vi "AIM_DataCollectAsCSV.vi"(5 "Data Reset?":bool, 7 "WRITE":bool, 10 "in X, Y Data":dbl[][](array[numeric]), 11 "Data File Name":string="Sample-Robot-2-Trajectory-TrajLibrary.csv") -> (0 "Y, X Pairs":T1[](array[typedef]) {"Y" format="%_7f"; "X" format="%_7f"}, 1 "X, Y Pairs":T1[](array[typedef]) {"Y" format="%_7f"; "X" format="%_7f"}, 2 "all Data":dbl[][](array[numeric]), 3 "Data File Name":string="Sample-Robot-2-Trajectory-TrajLibrary.csv")   [LabVIEW 2023]
uses:
  <vilib>/Rock Robotics/WPI/ThirdParty/JAS_Junk/TrajLib/TypeDef/X_Y_PAIR.ctl
  <vilib>/Utility/file.llb/Read Delimited Spreadsheet (DBL).vi
  <vilib>/Utility/file.llb/Write Delimited Spreadsheet (DBL).vi
  <vilib>/Rock Robotics/WPI/ThirdParty/JAS_Junk/TrajLib/Trajectory_Library.lvlib
panel:
  out "error out":errorcluster
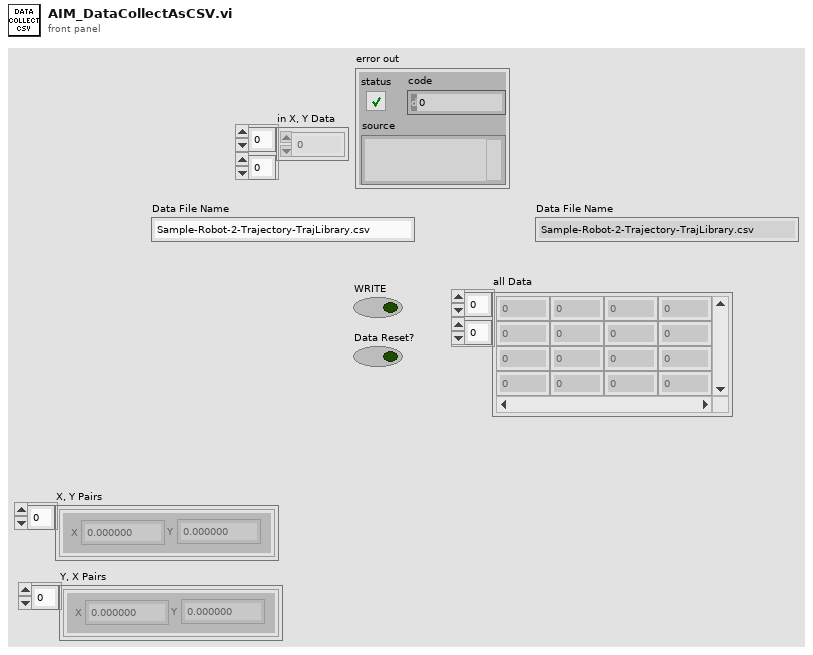
[diagram p1: front panel]
types:
  T1 = typedef "Trajectory_Library.lvlib/X_Y_PAIR.ctl" = cluster{"X":dbl, "Y":dbl}
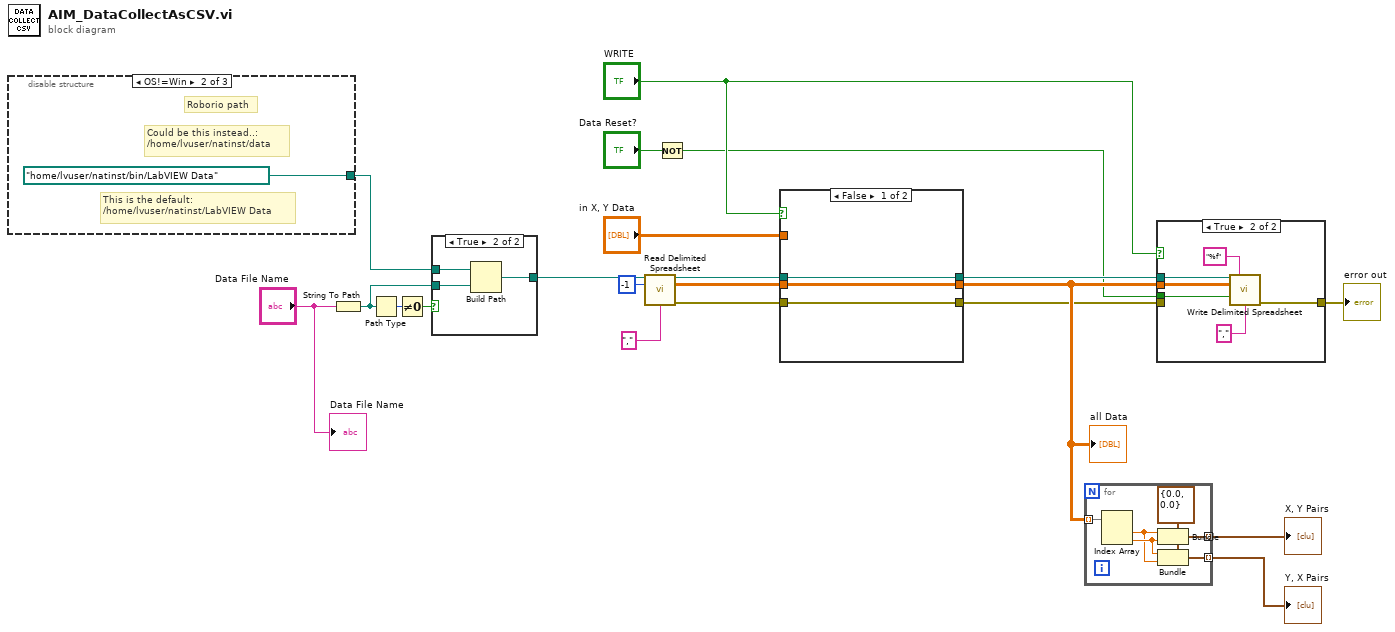
[diagram p0: block diagram]
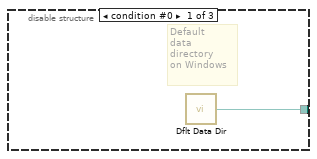
[diagram p4: hidden frame]
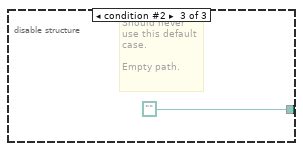
[diagram p5: hidden frame]
diagram:
  n1 = disable-structure shown="OS!=Win" {
    disable-tunnel: [w22 path "/home/lvuser/natinst/bin/LabVIEW Data" path ""] -> w19
    frame condition #0 {
      # "Default\ndata\ndirectory\non Windows"
      n2 = call <vilib>:"Dflt Data Dir.vi"() -> ("App:Default Data Directory"=w22:path)
    }
    frame condition #1 (active) {
      # "This is the default:\n/home/lvuser/natinst/LabVIEW Data"
      # "Could be this instead..:\n/home/lvuser/natinst/data"
      # "Roborio path"
    }
    frame condition #2 {
      # "Should never\nuse this default\ncase.\n\nEmpty path."
    }
  }
  n3 = String To Path(string="Data File Name") -> (path=w17:path)
  n4 = Path Type(1:w17) -> (0:w20:i16)
  n5 = Not Equal To 0?(x=w20) -> (x != 0?=w21:bool)
  n6 = case shown="True" w21 {
    tunnel: [w25 w28] -> w2
    tunnel: w19 -> [_ w27]
    tunnel: w17 -> [w25 w26]
    frame False {
    }
    frame True {
      n7 = Build Path(base path=w27, name or relative path=w26) -> (appended path=w28:path)
    }
  }
  n8 = call-poly <vilib>:"Read Delimited Spreadsheet.vi"("file path (dialog if empty)"=w2, "number of rows (all:-1)"=-1, "delimiter (\\t)"="," ("delimiter (\\t)")) -> ("new file path (Not A Path if cancelled)"=w1:path, "all rows"=w10:dbl[][], "error out"=w5:errorcluster)  [unwired: 7 in, 3 out]
  n9 = Not(x="Data Reset?") -> (.not. x?=w6:bool)
  n10 = case shown="False" "WRITE" {
    tunnel: w1 -> [w31 w34]
    tunnel: [w31 w34] -> w11
    tunnel: w10 -> [w30 _]
    tunnel: [w30 w33] -> w9
    tunnel: "in X, Y Data" -> [_ w33]
    tunnel: [w29 w32] -> w4
    tunnel: w5 -> [w29 w32]
    frame False {
    }
    frame True {
    }
  }
  "all Data" <- w9
  n11 = for {
    tunnel: w9 -> [w40] mode=indexing
    tunnel: [w39] -> w16 mode=indexing
    tunnel: [w35] -> w15 mode=indexing
    w37 = T1 {"X"=0.0, "Y"=0.0} ("X_Y_PAIR")
    n12 = Index Array(array=w40) -> (element #1=w36:dbl, element #2=w38:dbl)  [unwired: 2 in]
    n13 = Bundle(cluster=w37, "X"=w36, "Y"=w38) -> (w39:T1)
    n14 = Bundle(cluster=w37, "X"=w38, "Y"=w36) -> (w35:T1)
  }
  "X, Y Pairs" <- w16
  "Y, X Pairs" <- w15
  n15 = case shown="True" "WRITE" {
    tunnel: w9 -> [_ w47]
    tunnel: w11 -> [_ w46]
    tunnel: w6 -> [_ w43]
    tunnel: w4 -> [w41 _]
    tunnel: [w41 w42] -> w3
    frame False {
    }
    frame True {
      n16 = call-poly <vilib>:"Write Delimited Spreadsheet.vi"("file path (dialog if empty)"=w46, "format (%.3f)"="%f", "2D data"=w47, "append to file? (new file:F)"=w43, "delimiter (\\t)"="," ("delimiter (\\t)")) -> ("error out"=w42:errorcluster)  [unwired: 9 in, 1 out]
    }
  }
  "error out" <- w3
  "Data File Name" <- "Data File Name"
